vi "ep_Write Nominal Voltage.vi"(8 "error in (no error)":errorcluster, 10 "nominal voltage [V]":dbl=230.0, 11 "system info in":refnum<class "EP System Info.lvclass">) -> (0 "error out":errorcluster, 3 "system info out":refnum<class "EP System Info.lvclass">)   [LabVIEW 2014, in "NI_EP_Power Quality.lvlib" / "EP System Info.lvclass"]
uses:
  <vilib>/addons/Electrical Power/PQ/Common/Classes/System Info/EP System Info.lvclass
  <vilib>/addons/Electrical Power/PQ/Common/Classes/System Info/EP System Info.lvclass/EP System Info.ctl
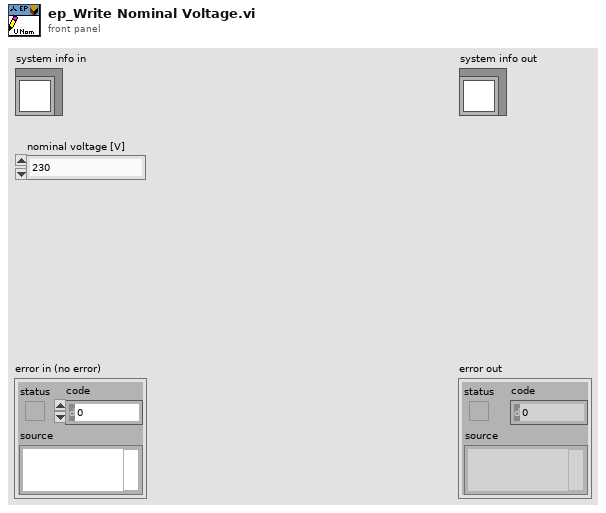
[diagram p1: front panel]
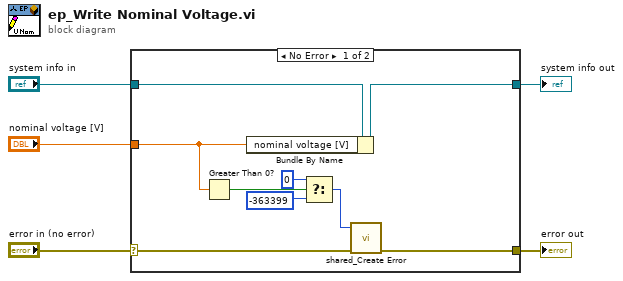
[diagram p0: block diagram]
diagram:
  n1 = case shown="No Error" "error in (no error)" {
    selector: "error in (no error)" -> [w7 w15]
    tunnel: [w6 w15] -> w4
    tunnel: [w13 w16] -> w2
    tunnel: "system info in" -> [w14 w16]
    tunnel: "nominal voltage [V]" -> [w12 _]
    frame No Error {
      n2 = Greater Than 0?(x=w12) -> (x > 0?=w8:bool)
      n3 = Bundle By Name(cluster=w14, "nominal voltage [V]"=w12) -> (w13:refnum<class "EP System Info.lvclass">)
      n4 = Select(t=0 ("upper limit"), s=w8, f=-363399 ("upper limit")) -> (s? t:f=w10:i32)
      n5 = call <vilib>:"shared_Create Error.vi"("error in (no error)"=w7, "error code (0)"=w10) -> ("error out"=w6:errorcluster)  [unwired: 9 in]
    }
    frame Error {
    }
  }
  "error out" <- w4
  "system info out" <- w2
